vi "Discrete Zero-Pole (DBL Array).vi"(2 "initialize":bool, 3 "Zeros-Poles-Gains":T1(array[cluster]) {"Poles" format="%.2f"; "Zeros" format="%.2f"; "gain" format="%.2f"}, 5 "input points":dbl[](array[numeric]) format="%.2f") -> (1 "Output points":dbl[](array[numeric]) format="%.2f")   [LabVIEW 2020, in "NI_AdvCtrl_discrete linear.lvlib"]
doc: "LabVIEW no longer supports this VI. You can obtain similar functionality by installing the LabVIEW Simulation Module.\n\nCalculates the new output point, where the discrete transfer function and the input point are given. The discrete transfer function is described in gain-zeros-poles notation."
uses:
  <vilib>/addons/control/advanced/NI_AdvCtrl_discrete linear.lvlib
  <vilib>/addons/control/advanced/NI_AdvCtrl_continuous linear.lvlib
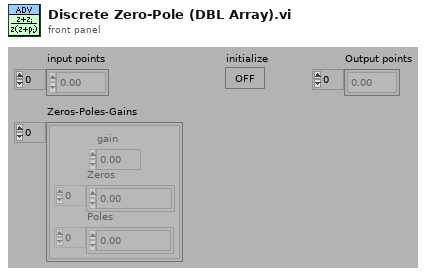
[diagram p1: front panel]
types:
  T1 = cluster{"gain":dbl, "Zeros":cdb[], "Poles":cdb[]}[]
  T2 = cluster{"Numerator new":dbl[], "Denominator new":dbl[]}[]
  T3 = cluster{"Numerator new":dbl[], "Denominator new":dbl[]}
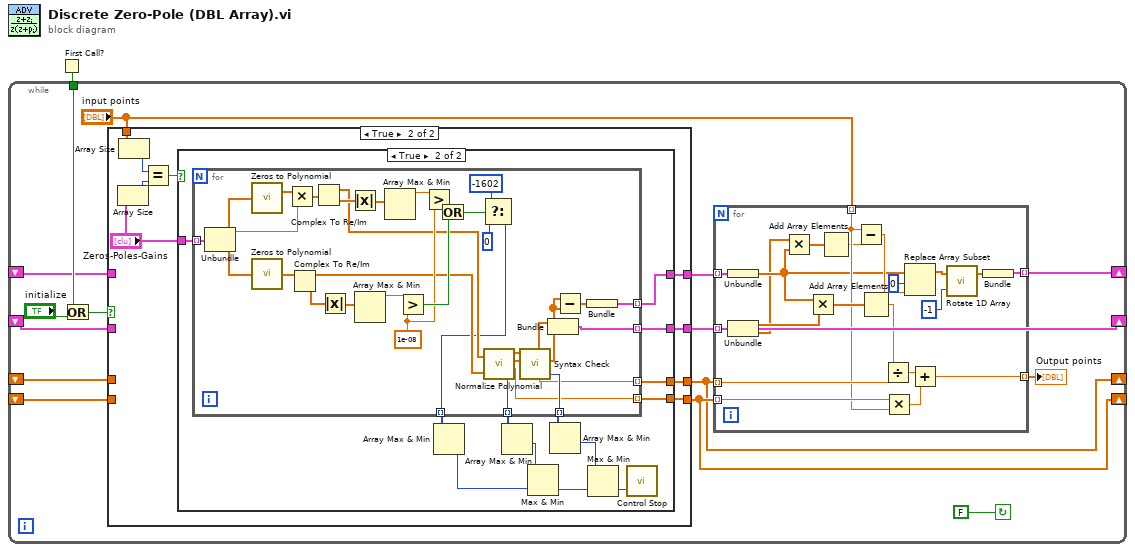
[diagram p0: block diagram]
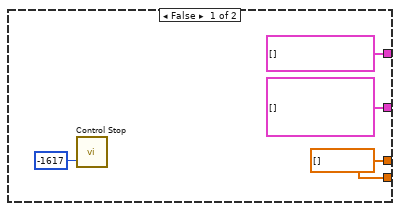
[diagram p3: hidden frame]
diagram:
  n1 = First Call?() -> (First Call?: T/F=w1:bool)
  n2 = while {
    shift-left: _ -> [w4]
    shift-right: [w5] -> _
    shift-left: _ -> [w7]
    shift-right: [w8] -> _
    tunnel: w1 -> [w10]
    shift-left: _ -> [w15]
    shift-right: [w14] -> _
    shift-left: _ -> [w16]
    shift-right: [w13] -> _
    stop <- FALSE continue-if-true
    n3 = Or(x=w10, y="initialize") -> (x .or. y?=w9:bool)
    n4 = case shown="True" w9 {
      tunnel: [w40 w50] -> w14
      tunnel: [w41 w49] -> w13
      tunnel: w16 -> [w41 _]
      tunnel: w15 -> [w40 _]
      tunnel: w7 -> [w38 _]
      tunnel: [w39 w48] -> w5
      tunnel: [w38 w47] -> w3
      tunnel: w4 -> [w39 _]
      tunnel: "input points" -> [_ w46]
      frame False {
      }
      frame True {
        n5 = Array Size(array="Zeros-Poles-Gains") -> (size(s)=w44:i32)
        n6 = Array Size(array=w46) -> (size(s)=w43:i32)
        n7 = Equal?(x=w43, y=w44) -> (x = y?=w42:bool)
        n8 = case shown="True" w42 {
          tunnel: [w52 w67] -> w50
          tunnel: [w52 w66] -> w49
          tunnel: "Zeros-Poles-Gains" -> [_ w65]
          tunnel: [T2 [] w64] -> w48
          tunnel: [cluster{dbl[]}[] [] w55] -> w47
          frame False {
            w52 = dbl[] []
            n9 = call <vilib>:"Control Stop.vi"("error"=-1617) -> ()  [unwired: 2 out]
          }
          frame True {
            n10 = for {
              tunnel: [w100] -> w62 mode=indexing
              tunnel: [w99] -> w63 mode=indexing
              tunnel: [w96] -> w67 mode=indexing
              tunnel: [w95] -> w66 mode=indexing
              tunnel: w65 -> [w79] mode=indexing
              tunnel: [w94] -> w64 mode=indexing
              tunnel: [w72] -> w61 mode=indexing
              tunnel: [w68] -> w55 mode=indexing
              w88 = 1e-08
              n11 = Unbundle(w79) -> ("gain"=w78:dbl, "Zeros"=w77:cdb[], "Poles"=w76:cdb[])
              n12 = call <vilib>:"Zeros to Polynomial.vi"("Zeros"=w77) -> ("Polynomial"=w84:cdb[])
              n13 = call <vilib>:"Zeros to Polynomial.vi"("Zeros"=w76) -> ("Polynomial"=w83:cdb[])
              n14 = Multiply(x=w84, y=w78) -> (x*y=w82:cdb[])
              n15 = Complex To Re/Im(x + iy=w83) -> (x=w81:dbl[], y=w86:dbl[])
              n16 = Complex To Re/Im(x + iy=w82) -> (x=w80:dbl[], y=w92:dbl[])
              n17 = Absolute Value(x=w86) -> (abs(x)=w85:dbl[])
              n18 = Absolute Value(x=w92) -> (abs(x)=w91:dbl[])
              n19 = Array Max & Min(array=w85) -> (max value=w87:dbl)  [unwired: 3 out]
              n20 = Array Max & Min(array=w91) -> (max value=w93:dbl)  [unwired: 3 out]
              n21 = Greater?(x=w87, y=w88) -> (0:w89:bool)
              n22 = Greater?(x=w93, y=w88) -> (0:w90:bool)
              n23 = Or(x=w90, y=w89) -> (x .or. y?=w75:bool)
              n24 = Select(t=-1602, s=w75, f=0) -> (s? t:f=w72:i32)
              n25 = call <vilib>:"Normalize Polynomial.vi"("Numerator"=w80, "Denominator"=w81) -> ("Numerator new"=w97:dbl[], "Denominator new"=w98:dbl[], "additive constant"=w96:dbl, "error"=w99:i32)
              n26 = call <vilib>:"Syntax Check.vi"("Denominator"=w98, "Numerator"=w97) -> ("error"=w100:i32, "gain"=w95:dbl, "Denominator new"=w70:dbl[], "Numerator new"=w71:dbl[])  [unwired: 1 out]
              n27 = Bundle("Numerator new"=w71, "Denominator new"=w70) -> (w94:T3)  [unwired: 1 out]
              n28 = Subtract(x=w70, y=w70) -> (x-y=w69:dbl[])
              n29 = Bundle(w69) -> (w68:cluster{dbl[]})  [unwired: 1 in]
            }
            n30 = Array Max & Min(array=w61) -> (min value=w59:i32)  [unwired: 3 out]
            n31 = Array Max & Min(array=w63) -> (min value=w60:i32)  [unwired: 3 out]
            n32 = Max & Min(x=w60, y=w59) -> (min(x,y)=w57:i32)  [unwired: 1 out]
            n33 = Array Max & Min(array=w62) -> (min value=w58:i32)  [unwired: 3 out]
            n34 = Max & Min(x=w58, y=w57) -> (min(x,y)=w56:i32)  [unwired: 1 out]
            n35 = call <vilib>:"Control Stop.vi"("error"=w56) -> ()  [unwired: 2 out]
          }
        }
      }
    }
    n36 = for {
      tunnel: w14 -> [w35] mode=indexing
      tunnel: w13 -> [w34] mode=indexing
      tunnel: [w20] -> w8 mode=indexing
      tunnel: w3 -> [w27] mode=indexing
      tunnel: "input points" -> [w30] mode=indexing
      tunnel: [w29] -> w6 mode=indexing
      tunnel: w5 -> [w24] mode=indexing
      n37 = Unbundle(w27) -> ("array (last n elements first)"=w22:dbl[])
      n38 = Unbundle(w24) -> ("Numerator new"=w23:dbl[], "Denominator new"=w21:dbl[])
      n39 = Multiply(x=w21, y=w22) -> (x*y=w26:dbl[])
      n40 = Multiply(x=w22, y=w23) -> (x*y=w32:dbl[])
      n41 = Add Array Elements(numeric array=w26) -> (sum=w25:dbl)
      n42 = Subtract(x=w30, y=w25) -> (x-y=w33:dbl)
      n43 = Add Array Elements(numeric array=w32) -> (sum=w31:dbl)
      n44 = Divide(x=w31, y=w34) -> (x/y=w36:dbl)
      n45 = Multiply(x=w35, y=w30) -> (x*y=w37:dbl)
      n46 = Replace Array Subset(array=w22, new element=w33, index=0 ("Index")) -> (w18:dbl[])
      n47 = Add(x=w36, y=w37) -> (x+y=w29:dbl)
      n48 = call <vilib>:"Rotate 1D Array.vi"("n"=-1, "array"=w18) -> ("array (last n elements first)"=w19:dbl[])  [unwired: 1 out]
      n49 = Bundle("array (last n elements first)"=w19) -> (w20:cluster{"array (last n elements first)":dbl[]})  [unwired: 1 in]
    }
    "Output points" <- w6
  }
